vi "WriteOperatingStates.vi"(8 "error in (no error)":errorcluster, 11 "body":u8[](array[numeric])) -> (0 "error out":errorcluster)   [LabVIEW 2017, in "ServerComm.lvlib"]
uses:
  <vilib>/addons/InsightCM/Devices/Shared/Common/ServerComm/ServerComm.lvlib
  <vilib>/addons/InsightCM/MessageBus/Base/controls/ConfigListItem.ctl
  <vilib>/addons/InsightCM/Utilities/GlobalConfiguration/GlobalConfiguration.lvlib
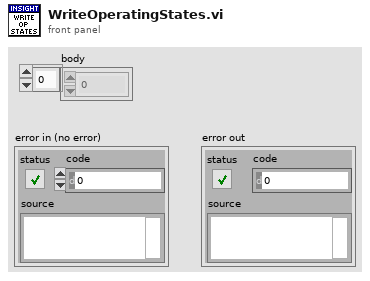
[diagram p1: front panel]
types:
  T1 = typedef "ConfigListItem.ctl" = cluster{"Id":string, "Name":string, "ReadOnly":bool, "Weight":i32}
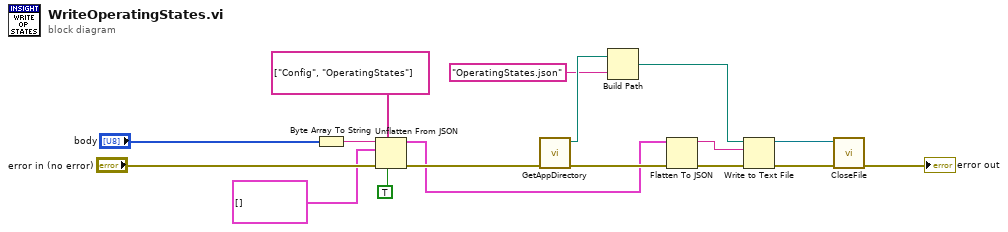
[diagram p0: block diagram]
diagram:
  n1 = Byte Array To String(unsigned byte array="body") -> (string=w7:string)
  n2 = Unflatten From JSON(path=string[] ["Config", "OperatingStates"], JSON string=w7, type and defaults=T1[] [] ("OperatingStates"), default null elements? (F)=TRUE, error in (no error)="error in (no error)") -> (value=w1:T1[], error out=w3:errorcluster)  [unwired: 2 in]
  n3 = call <vilib>:"GetAppDirectory.vi"("error in (no error)"=w3) -> ("error out"=w15:errorcluster, "application directory"=w17:path)  [unwired: 9 in]
  n4 = Build Path(base path=w17, name or relative path="OperatingStates.json") -> (appended path=w13:path)
  n5 = Flatten To JSON(anything=w1, error in (no error)=w15) -> (JSON string=w12:string, 11:w14:errorcluster)  [unwired: 1 in]
  n6 = Write to Text File(file (use dialog)=w13, text=w12, error in=w14) -> (refnum out=w11:refnum<file>, error out=w10:errorcluster)  [unwired: 1 in, 1 out]
  n7 = call <vilib>:"CloseFile.vi"("error in (no error)"=w10, "file reference"=w11) -> ("error out"=→"error out":errorcluster)  [unwired: 9 in]
